vi "StopFiltering.vi"(8 "error in":errorcluster, 11 "SubPanel in":refnum<vi>) -> (0 "error out":errorcluster, 2 "StopAck":bool)   [LabVIEW 2013, in "FindName Task_Manager.lvlib"]
uses:
  FindName Task_Manager.lvlib
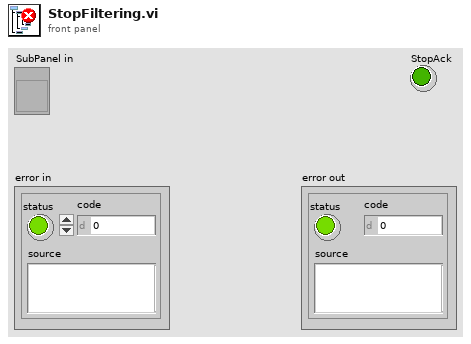
[diagram p1: front panel]
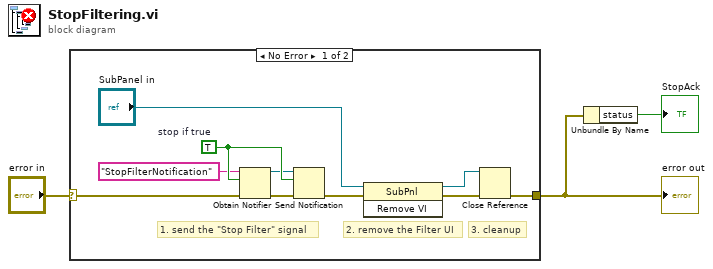
[diagram p0: block diagram]
diagram:
  n1 = case shown="No Error" "error in" {
    selector: "error in" -> [w6 w14]
    tunnel: [w5 w14] -> w2
    frame No Error {
      w12 = TRUE  # stop if true
      # "3. cleanup"
      # "2. remove the Filter UI"
      # "1. send the \"Stop Filter\" signal"
      n2 = Obtain Notifier(name (unnamed)="StopFilterNotification", notification data type=w12, error in (no error)=w6) -> (notifier out=w9:refnum<notifier>, error out=w10:errorcluster)  [unwired: 1 in, 1 out]
      n3 = Send Notification(notification=w12, notifier=w9, error in (no error)=w10) -> (error out=w11:errorcluster)  [unwired: 1 out]
      n4 = invoke on="Invoke Node" class="SubPnl" method="Remove VI"(reference="SubPanel in", error in=w11) -> (reference out=w4:refnum<vi>, error out=w13:errorcluster)  [unwired: 1 in, 1 out]
      n5 = Close Reference(reference=w4, error in (no error)=w13) -> (error out=w5:errorcluster)
    }
    frame Error {
    }
  }
  "error out" <- w2
  n6 = Unbundle By Name(w2) -> ("status"=→"StopAck":bool)
